vi "Climb_Teleop.vi"(11 "Joystick_In":T1) -> ()   [LabVIEW 2019]
uses:
  Climb_Pivot/Climb_Pivot_Control_States.ctl
  Climb_Pivot/Climb_Pivot_Cluster.ctl
  Climb_Elevator/Climb_Elevator_Control_States.ctl
  Climb_Elevator/Climb_Elevator_Cluster.ctl
  Climb_Transverse/Climb_Transverse_Control_States.ctl
  Climb_Transverse/Climb_Transverse_Cluster.ctl
  Climb_Globals.vi
  Utility_VIs/Joystick_Controls.ctl
panel:
  in  "transverse_power":dbl=1.0
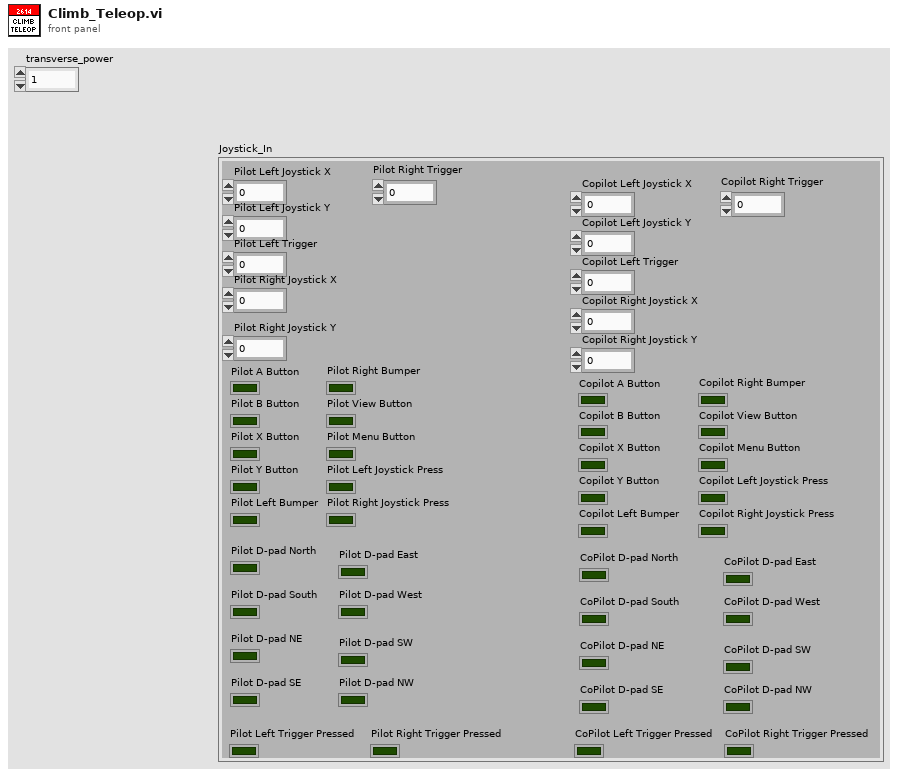
[diagram p1: front panel]
types:
  T1 = typedef "Joystick_Controls.ctl" = cluster{"Pilot Left Joystick X":dbl, "Pilot Left Joystick Y":dbl, "Pilot A Button":bool, "Pilot B Button":bool, "Pilot X Button":bool, "Pilot Y Button":bool, "Pilot Left Bumper":bool, "Pilot Right Bumper":bool, "Pilot View Button":bool, "Pilot Menu Button":bool, "Pilot Left Joystick Press":bool, "Pilot Right Joystick Press":bool, "Pilot Left Trigger":dbl, "Pilot Right Joystick X":dbl, "Pilot Right Joystick Y":dbl, "Pilot Right Trigger":dbl, "Copilot Left Joystick X":dbl, "Copilot Left Joystick Y":dbl, "Copilot A Button":bool, "Copilot B Button":bool, "Copilot X Button":bool, "Copilot Y Button":bool, "Copilot Left Bumper":bool, "Copilot Right Bumper":bool, "Copilot View Button":bool, "Copilot Menu Button":bool, "Copilot Left Joystick Press":bool, "Copilot Right Joystick Press":bool, "Copilot Left Trigger":dbl, "Copilot Right Joystick X":dbl, "Copilot Right Joystick Y":dbl, "Copilot Right Trigger":dbl, "Pilot D-pad North":bool, "Pilot D-pad South":bool, "Pilot D-pad East":bool, "Pilot D-pad West":bool, "Pilot D-pad NE ":bool, "Pilot D-pad SE":bool, "Pilot D-pad SW":bool, "Pilot D-pad NW":bool, "CoPilot D-pad North":bool, "CoPilot D-pad South":bool, "CoPilot D-pad East":bool, "CoPilot D-pad West":bool, "CoPilot D-pad NE":bool, "CoPilot D-pad SE":bool, "CoPilot D-pad SW":bool, "CoPilot D-pad NW":bool, "Pilot Left Trigger Pressed":bool, "Pilot Right Trigger Pressed":bool, "CoPilot Left Trigger Pressed":bool, "CoPilot Right Trigger Pressed":bool}
  T2 = typedef "Climb_Transverse_Cluster.ctl" = cluster{"Auto-Balance?":bool, "Transverse_Throttle":dbl, "Control_States":T3}
  T3 = typedef "Climb_Transverse_Control_States.ctl" = enum16{"No-Op", "Manual", "Auto-Balancing"}
  T4 = typedef "Climb_Elevator_Cluster.ctl" = cluster{"Extend?":bool, "Elevator_Throttle":dbl, "Control_States":T5, "Brake?":bool}
  T5 = typedef "Climb_Elevator_Control_States.ctl" = enum16{"No-Op", "Brake", "Going_Up", "Going_Down", "Manual_PercentVoltage", "Manual_SpeedControl"}
  T6 = typedef "Climb_Pivot_Cluster.ctl" = cluster{"Up?":bool, "Pivot_Throttle":dbl, "Control_States":T7}
  T7 = typedef "Climb_Pivot_Control_States.ctl" = enum16{"No-Op", "Moving_Down", "Moving_Up", "Manual"}
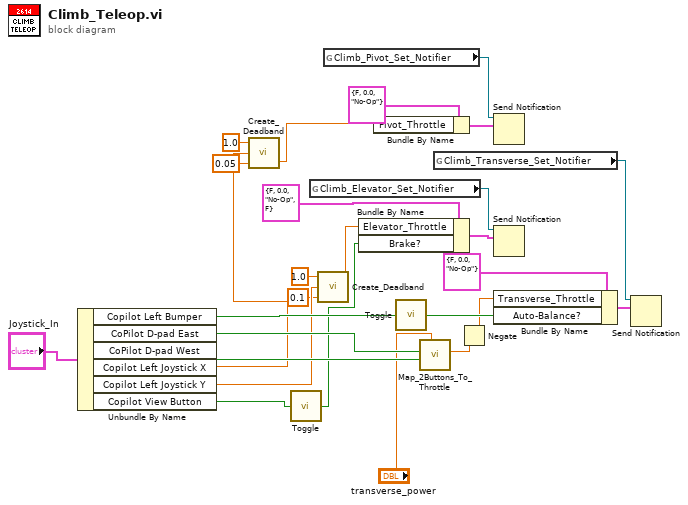
[diagram p0: block diagram]
diagram:
  n1 = Unbundle By Name("Joystick_In") -> ("Copilot Left Bumper"=w26:bool, "CoPilot D-pad East"=w15:bool, "CoPilot D-pad West"=w14:bool, "Copilot Left Joystick X"=w10:dbl, "Copilot Left Joystick Y"=w6:dbl, "Copilot View Button"=w2:bool)
  n2 = call "Create_Deadband.vi"("Output Lower Limit"=0.05, "Input"=w10, "Output Upper Limit"=1.0) -> ("Output"=w11:dbl)  [unwired: 1 out]
  n3 = call "Toggle.vi"("Boolean"=w2) -> ("Boolean Out"=w1:bool)
  n4 = global read "Climb_Globals.vi" "Climb_Elevator_Set_Notifier"() -> (w20:refnum<notifier>)
  n5 = call "Create_Deadband.vi"("Output Lower Limit"=0.1, "Input"=w6, "Output Upper Limit"=1.0) -> ("Output"=w7:dbl)  [unwired: 1 out]
  n6 = global read "Climb_Globals.vi" "Climb_Pivot_Set_Notifier"() -> (w21:refnum<notifier>)
  n7 = Bundle By Name(cluster=T4 {"Extend?"=FALSE, "Elevator_Throttle"=0.0, "Control_States"=enum."No-Op", "Brake?"=FALSE} ("Climb_Pivot_Cluster"), "Elevator_Throttle"=w7, "Brake?"=w1) -> (w19:T4)
  n8 = Bundle By Name(cluster=T6 {"Up?"=FALSE, "Pivot_Throttle"=0.0, "Control_States"=enum."No-Op"} ("Climb_Pivot_Cluster"), "Pivot_Throttle"=w11) -> (w22:T6)
  n9 = call "Toggle.vi"("Boolean"=w26) -> ("Boolean Out"=w16:bool)
  n10 = call "Map_2Buttons_To_Throttle.vi"("Power"="transverse_power", "Down"=w14, "Up"=w15) -> ("Throttle"=w12:dbl)  [unwired: 8 in]
  n11 = global read "Climb_Globals.vi" "Climb_Transverse_Set_Notifier"() -> (w18:refnum<notifier>)
  n12 = Negate(x=w12) -> (-x=w3:dbl)
  n13 = Send Notification(notification=w22, notifier=w21) -> ()  [unwired: 1 in, 2 out]
  n14 = Send Notification(notification=w19, notifier=w20) -> ()  [unwired: 1 in, 2 out]
  n15 = Bundle By Name(cluster=T2 {"Auto-Balance?"=FALSE, "Transverse_Throttle"=0.0, "Control_States"=enum."No-Op"} ("Climb_Transverse_Cluster"), "Transverse_Throttle"=w3, "Auto-Balance?"=w16) -> (w17:T2)
  n16 = Send Notification(notification=w17, notifier=w18) -> ()  [unwired: 1 in, 2 out]
